vi "Set Data Call Alg Get Data.vi"(4 "QWTB Folder Path":path=path "", 5 "Calculation Settings":T2={"Verbose"=FALSE, "Uncertainty Calculation Method"=enum."none", "Correlations"={"Required"=FALSE, "Generate"=TRUE}, "Degrees of Freedom"={"Required"=FALSE, "Generate"=FALSE}, "MCM Calculation Settings"={"Repeats"=100, "Verbose"=TRUE, "Parallelization method"=enum."Single Core", "Processors"=1, "Temporary directory"=".", "Randomize"=TRUE}} {"MCM Calculation Settings"."Processors" min=1 step=1; "MCM Calculation Settings"."Repeats" min=1 step=1}, 6 "Backend engine":T1, 7 "Algorithm Information":T9, 8 "error in":errorcluster, 11 "Data In":T8[](array[typedef])) -> (0 "error out":errorcluster, 3 "Data Out":T8[](array[typedef]))   [LabVIEW 2013]
doc: "Clears Matlab variables, set working path, writes input data, writes calculation settings, calls algorithm, reads output data."
uses:
  TD Algorithm Information.ctl
  TD Quantity.ctl
  TD Calculation Settings.ctl
  TD Uncertainty Calculation Method.ctl
  TD Correlation Calculation Settings.ctl
  TD DOF Calculation Settings.ctl
  TD MCM Calculation Settings.ctl
  TD MCM Calculation Method.ctl
  TD Backend Engine.ctl
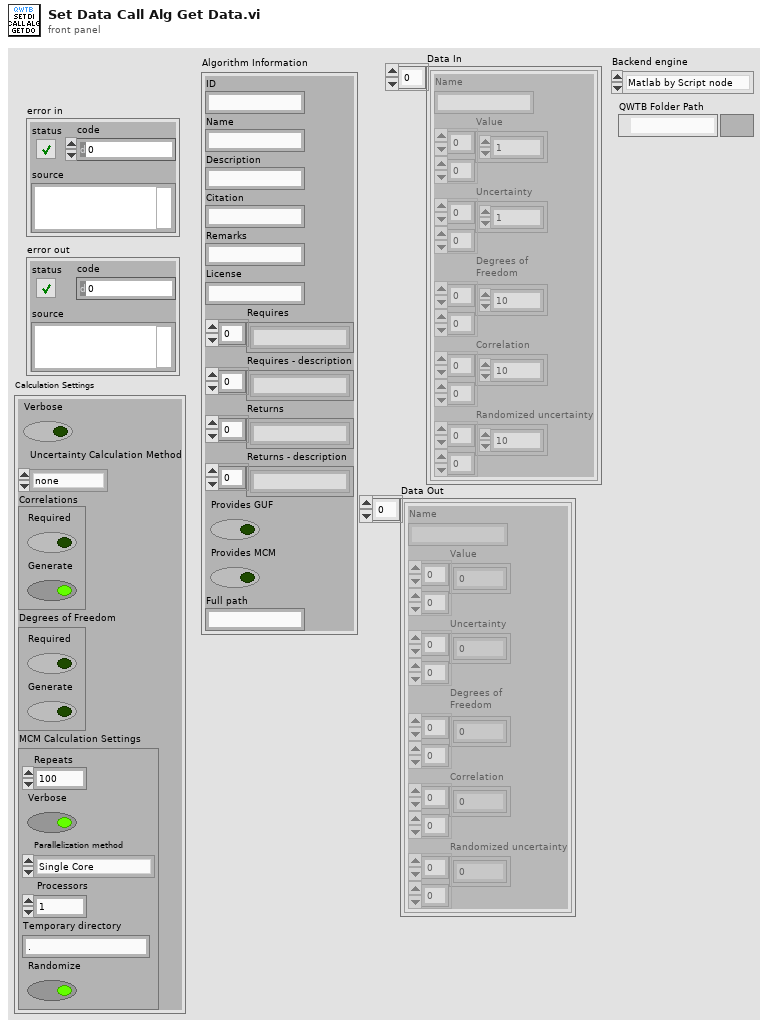
[diagram p1: front panel]
types:
  T1 = typedef "TD Backend Engine.ctl" = enum16{"Matlab by Script node", "GNU Octave by GOLPI"}
  T2 = typedef "TD Calculation Settings.ctl" = cluster{"Verbose":bool, "Uncertainty Calculation Method":T3, "Correlations":T4, "Degrees of Freedom":T5, "MCM Calculation Settings":T6}
  T3 = typedef "TD Uncertainty Calculation Method.ctl" = enum16{"none", "GUF", "MCM"}
  T4 = typedef "TD Correlation Calculation Settings.ctl" = cluster{"Required":bool, "Generate":bool}
  T5 = typedef "TD DOF Calculation Settings.ctl" = cluster{"Required":bool, "Generate":bool}
  T6 = typedef "TD MCM Calculation Settings.ctl" = cluster{"Repeats":i32, "Verbose":bool, "Parallelization method":T7, "Processors":i32, "Temporary directory":string, "Randomize":bool}
  T7 = typedef "TD MCM Calculation Method.ctl" = enum16{"Single Core", "Multi Core", "Multi Station"}
  T8 = typedef "TD Quantity.ctl" = cluster{"Name":string, "Value":dbl[][], "Uncertainty":dbl[][], "Degrees of\nFreedom":dbl[][], "Correlation":dbl[][], "Randomized uncertainty":dbl[][]}
  T9 = typedef "TD Algorithm Information.ctl" = cluster{"ID":string, "Name":string, "Description":string, "Citation":string, "Remarks":string, "License":string, "Requires":string[], "Requires - description":string[], "Returns":string[], "Returns - description":string[], "Provides GUF":bool, "Provides MCM":bool, "Full path":string}
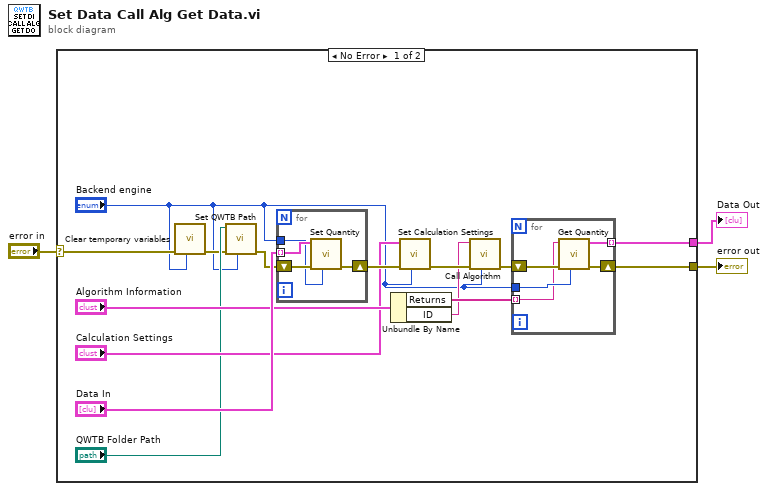
[diagram p0: block diagram]
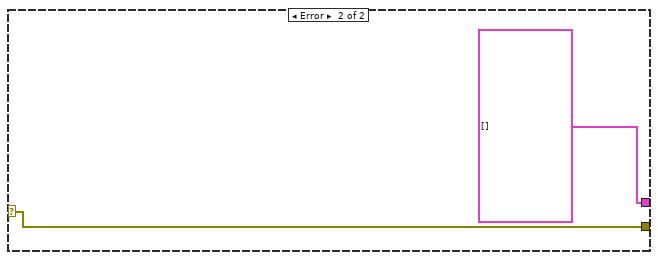
[diagram p2: hidden frame]
diagram:
  n1 = case shown="No Error" "error in" {
    selector: "error in" -> [w5 w29]
    tunnel: [w15 w29] -> w3
    tunnel: [w8 T8[] []] -> w1
    frame No Error {
      n2 = call "Clear temporary variables.vi"("Backend engine"="Backend engine", "error in"=w5) -> ("error out"=w6:errorcluster)  [unwired: 9 in]
      n3 = call "Set QWTB Path.vi"("Backend engine"="Backend engine", "error in"=w6, "QWTB Folder Path"="QWTB Folder Path") -> ("error out"=w11:errorcluster)  [unwired: 8 in]
      n4 = for {
        tunnel: "Data In" -> [w27] mode=indexing
        shift-right: [w25] -> w14
        shift-left: w11 -> [w26]
        tunnel: "Backend engine" -> [w24]
        n5 = call "Set Quantity.vi"("Backend engine"=w24, "error in"=w26, "Quantity"=w27) -> ("error out"=w25:errorcluster)  [unwired: 8 in]
      }
      n6 = Unbundle By Name("Algorithm Information") -> ("Returns"=w10:string[], "ID"=w9:string)
      n7 = call "Set Calculation Settings.vi"("Backend engine"="Backend engine", "error in"=w14, "Calculation Settings"="Calculation Settings") -> ("error out"=w13:errorcluster)  [unwired: 8 in]
      n8 = call "Call Algorithm.vi"("Backend engine"="Backend engine", "error in"=w13, "Algorithm ID"=w9) -> ("error out"=w16:errorcluster)  [unwired: 8 in]
      n9 = for {
        shift-right: [w22] -> w15
        shift-left: w16 -> [w23]
        tunnel: [w21] -> w8 mode=indexing
        tunnel: w10 -> [w19] mode=indexing
        tunnel: "Backend engine" -> [w20]
        n10 = call "Get Quantity.vi"("Backend engine"=w20, "error in"=w23, "Quantity Name"=w19) -> ("error out"=w22:errorcluster, "Quantity"=w21:T8)  [unwired: 7 in]
      }
    }
    frame Error {
    }
  }
  "error out" <- w3
  "Data Out" <- w1
